vi "Example.vi"() -> ()   [LabVIEW 2012]
uses:
  Polymorph Write Registers/EtherNet CIP WriteBit.vi
  Polymorph Write Registers/EtherNet CIP WriteReal_Array.vi
  Polymorph Write Registers/EtherNet CIP WriteINT_Array.vi
  Polymorph Read Registers/EtherNet CIP ReadBit.vi
  Polymorph Read Registers/EtherNet CIP ReadReal_Array.vi
  Polymorph Read Registers/EtherNet CIP ReadINT_Array.vi
panel:
  out "?":errorcluster
  in  "Read/\nWrite":bool
  in  "?":bool
  out "INT \nRead":u16[](array[numeric])
  in  "INT \nWrite":u16[](array[numeric])
  out "REAL \nRead":sgl[](array[numeric])
  in  "REAL \nWrite":sgl[](array[numeric])
  out "BOOL \nRead":bool
  in  "BOOL\nWrite":bool
  in  "Tag Bit":string
  in  "Tag Integer":string
  in  "Tag Real":string
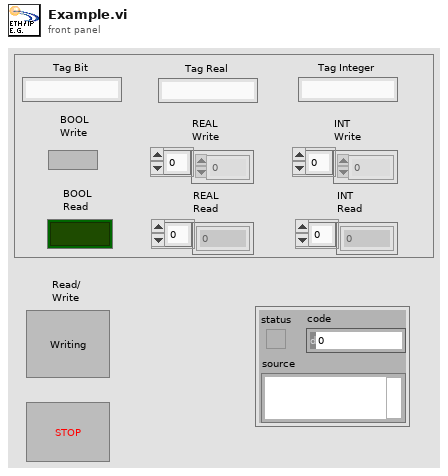
[diagram p1: front panel]
types:
  T1 = cluster{"TCP Connection":refnum<k5>, "Session":u8[], "EtherNet/IP Device Address":string}
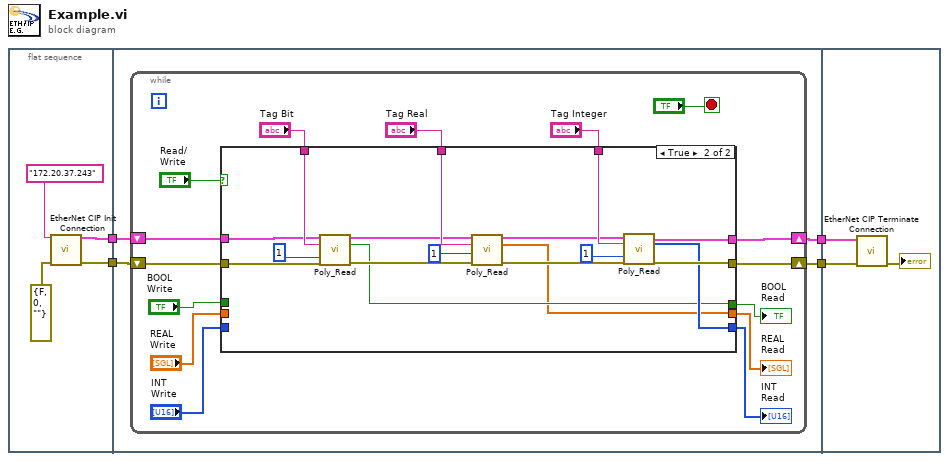
[diagram p0: block diagram]
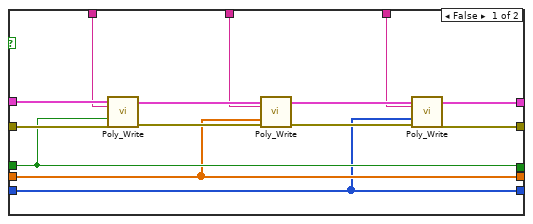
[diagram p2: hidden frame]
diagram:
  n1 = flat-sequence {
    tunnel: [w8] -> w4
    tunnel: [w5] -> w3
    tunnel: w4 -> [w12]
    tunnel: w3 -> [w9]
    tunnel: [w11] -> w2
    tunnel: [w10] -> w1
    tunnel: w2 -> [w61]
    tunnel: w1 -> [w60]
    frame #0 {
      n2 = call "EtherNet CIP Init Connection.vi"("EtherNet/IP Device Address"="172.20.37.243", "error in"=errorcluster {"status"=FALSE, "code"=0, "source"=""}) -> ("Connection Cluster"=w8:T1, "error out"=w5:errorcluster)  [unwired: 12 in]
    }
    frame #1 {
      n3 = while {
        shift-right: [w27] -> w11
        shift-left: w12 -> [w24]
        shift-right: [w26] -> w10
        shift-left: w9 -> [w25]
        stop <- "?" stop-if-true
        n4 = case shown="True" "Read/\nWrite" {
          tunnel: w24 -> [w35 w48]
          tunnel: w25 -> [w34 w58]
          tunnel: [w37 w44] -> w27
          tunnel: [w36 w56] -> w26
          tunnel: "Tag Bit" -> [w33 w54]
          tunnel: "Tag Real" -> [w32 w51]
          tunnel: "Tag Integer" -> [w31 w50]
          tunnel: "BOOL\nWrite" -> [w30 _]
          tunnel: "REAL \nWrite" -> [w29 _]
          tunnel: [w29 w42] -> w18
          tunnel: [w28 w45] -> w16
          tunnel: "INT \nWrite" -> [w28 _]
          tunnel: [w30 w43] -> w13
          frame False {
            n5 = call-poly "Poly_Write.vi"("Connection Cluster"=w35, "Tag"=w33, "BOOL"=w30, "error in"=w34) -> ("Connection Cluster Out"=w40:T1, "error out"=w39:errorcluster)  [unwired: 10 in]
            n6 = call-poly "Poly_Write.vi"("Connection Cluster"=w40, "Tag"=w32, "REAL Array"=w29, "error in"=w39) -> ("Connection Cluster Out"=w41:T1, "error out"=w38:errorcluster)  [unwired: 10 in]
            n7 = call-poly "Poly_Write.vi"("Connection Cluster"=w41, "Tag"=w31, "INT Array"=w28, "error in"=w38) -> ("Connection Cluster Out"=w37:T1, "error out"=w36:errorcluster)  [unwired: 10 in]
          }
          frame True {
            n8 = call-poly "Poly_Read.vi"("Connection Cluster"=w48, "Tag"=w54, "No of Elements"=u8 1, "error in"=w58) -> ("Connection Cluster out"=w46:T1, "BOOL"=w43:bool, "error out"=w57:errorcluster)  [unwired: 9 in]
            n9 = call-poly "Poly_Read.vi"("Connection Cluster"=w46, "Tag"=w51, "No of Elements"=u8 1, "error in"=w57) -> ("Connection Cluster Out"=w47:T1, "REAL Array"=w42:sgl[], "error out"=w55:errorcluster)  [unwired: 9 in]
            n10 = call-poly "Poly_Read.vi"("Connection Cluster"=w47, "Tag"=w50, "Num of Elements"=u8 1 ("No of Elements"), "error in"=w55) -> ("Connection Cluster Out"=w44:T1, "INT Array"=w45:u16[], "error out"=w56:errorcluster)  [unwired: 9 in]
          }
        }
        "BOOL \nRead" <- w13
        "REAL \nRead" <- w18
        "INT \nRead" <- w16
      }
    }
    frame #2 {
      n11 = call "EtherNet CIP Terminate Connection.vi"("Connection Cluster"=w61, "error in"=w60) -> ("error out"=→"?":errorcluster)  [unwired: 13 in]
    }
  }
